vi "Get Connections - 1Pin 1Conn.vi"(6 "pin type":T3, 8 "error in":errorcluster, 9 "site":i32, 10 "pin or relay name":string, 11 "session reservation in":refnum<class "Session Reservation.lvclass">) -> (0 "error out":errorcluster, 2 "connection":T1, 3 "session reservation out":refnum<class "Session Reservation.lvclass">)   [LabVIEW 2021, in "Session Management niSwitch.lvlib"]
doc: "Gets the NI-Switch connection information for the given <b>pin type</b>, <b>pin or relay name</b>, and <b>site</b>. If the <b>pin or relay name</b> input is unwired, the connection information for all pins on the given <b>site</b> will be returned. If the <b>site</b> input is unwired, the connection information for the given <b>pin or relay name</b> for all sites will be returned. If both the <b>pin or relay name</b> and <b>site</b> inputs are unwired, the connection information for all pins and on all sites will be returned.\n\nThe <b>pin type</b> input determines what type of pins to get: DUT pins, system pins, or all pins. \n\nIf you have not called <b>Initialize Sessions.vi</b> prior to calling this VI, the connection information will be returned with the correct information but will have an invalid session.\n\nThis VI returns an error if multiple connections match the inputs. Use <b>Get Connections - 1Pin MConn.vi</b> to get multiple connections from a single pin."
uses:
  Session Management niSwitch.lvlib
  <vilib>/Plug-In SDKs/Clients/Session Management V1/Session Reservation/Pin Type.ctl
  <vilib>/Plug-In SDKs/Clients/Session Management V1/Session Reservation/Session Reservation.lvclass
  Connection with Session.ctl
  Session Factory/Session Factory.lvclass
  C:/Program Files/National Instruments/LabVIEW 2021/vi.lib/Plug-In SDKs/Sessions/Instrument/ISession Factory/ISession Factory.lvclass
  <vilib>/Plug-In SDKs/Clients/Session Management V1/Session Reservation/Connection.ctl
  cf13ef01-879f-4978-ad5d-95f52dc7dba6.vi
  cf13ef01-879f-4978-ad5d-95f52dc7dba6.vi/d089b476-b30c-4b91-b2ff-fbae0086b065.vi
  <vilib>/Plug-In SDKs/Clients/Session Management V1/Session Reservation/Pin to Pin Array.vi
  <vilib>/Plug-In SDKs/Clients/Session Management V1/Session Reservation/Get Connections Impl.vi
  <vilib>/Plug-In SDKs/Measurements/Helpers/Error Strings Global Internal.vi
  <vilib>/Utility/error.llb/Error Cluster From Error Code.vi
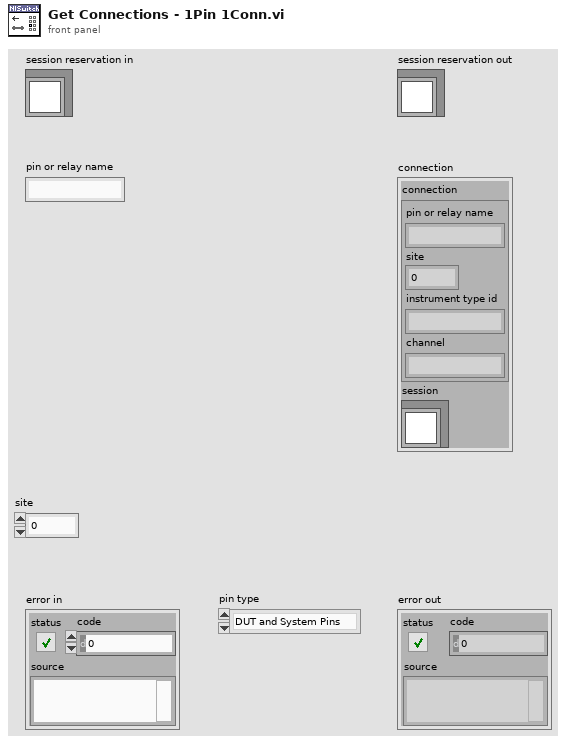
[diagram p1: front panel]
types:
  T1 = typedef "Session Management niSwitch.lvlib/Connection with Session.ctl" = cluster{"connection":T2, "session":refnum<class "Session Factory.lvclass">}
  T2 = typedef "NI Session Management V1 Client.lvlib/Session Reservation.lvclass/Connection.ctl" = cluster{"pin or relay name":string, "site":i32, "instrument type id":string, "channel":string}
  T3 = typedef "NI Session Management V1 Client.lvlib/Session Reservation.lvclass/Pin Type.ctl" = enum16{"DUT and System Pins", "System Pins"}
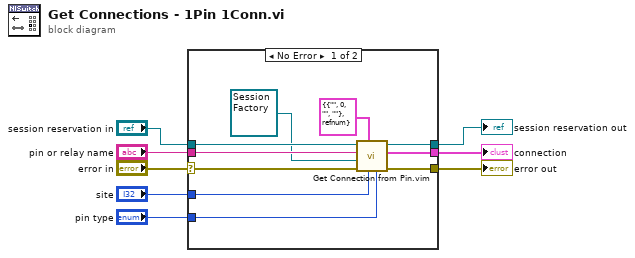
[diagram p0: block diagram]
diagram:
  n1 = case shown="No Error" "error in" {
    selector: "error in" -> [w16 w20]
    tunnel: "site" -> [w18 _]
    tunnel: "pin type" -> [w17 _]
    tunnel: [w15 w20] -> w5
    tunnel: "pin or relay name" -> [w14 _]
    tunnel: "session reservation in" -> [w13 w19]
    tunnel: [w12 w19] -> w2
    tunnel: [w9 _] -> w1
    frame No Error {
      n2 = call "Get Connection from Pin.vim"("pin type"=w17, "site"=w18, "connection type"=T1 {"connection"={"pin or relay name"="", "site"=0, "instrument type id"="", "channel"=""}, "session"=refnum} ("connection with task"), "error in"=w16, "session factory"=refnum<class "Session Factory.lvclass"> refnum ("Session Management niSwitch.lvlib:Session Factory.lvclass"), "pin or relay name"=w14, "session reservation in"=w13) -> ("error out"=w15:errorcluster, "connection"=w9:T1, "session reservation out"=w12:refnum<class "Session Reservation.lvclass">)  [unwired: 2 in]
    }
    frame Error {
    }
  }
  "error out" <- w5
  "session reservation out" <- w2
  "connection" <- w1
